vi "interp_3d.vi"(0 "prelookup_x":cluster{"frac":dbl, "num":u8}, 1 "prelookup_y":cluster{"frac":dbl, "num":u8}, 2 "z":dbl[][](array[numeric])) -> (7 "z":dbl)   [LabVIEW 2013]
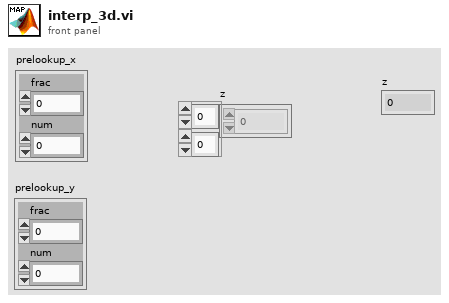
[diagram p1: front panel]
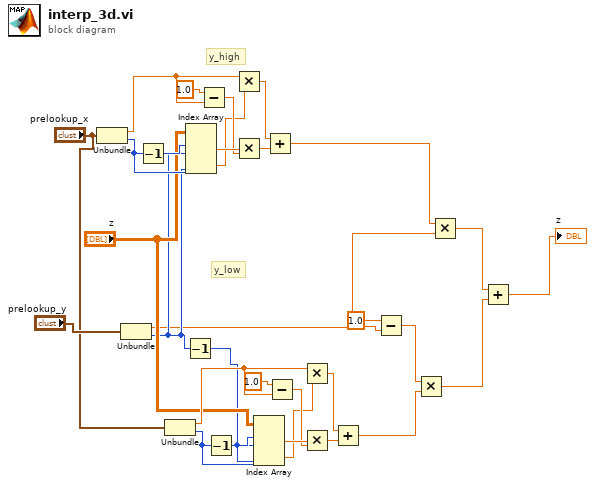
[diagram p0: block diagram]
diagram:
  # "y_low"
  # "y_high"
  n1 = Unbundle("prelookup_x") -> ("frac"=w30:dbl, "num"=w26:u8)
  n2 = Unbundle("prelookup_y") -> ("frac"=w2:dbl, "num"=w5:u8)
  n3 = Decrement(x=w26) -> (x-1=w27:u8)
  n4 = Unbundle("prelookup_x") -> ("frac"=w20:dbl, "num"=w16:u8)
  n5 = Decrement(x=w5) -> (x-1=w4:u8)
  n6 = Index Array(array="z", index (row) #1=w27, index (col) #1=w5, index (row) #2=w26, index (col) #2=w5) -> (element #1=w25:dbl, element #2=w23:dbl)
  n7 = Subtract(x=1.0, y=w30) -> (x-y=w24:dbl)
  n8 = Decrement(x=w16) -> (x-1=w17:u8)
  n9 = Multiply(x=w30, y=w23) -> (x*y=w29:dbl)
  n10 = Multiply(x=w25, y=w24) -> (x*y=w28:dbl)
  n11 = Index Array(array="z", index (row) #1=w17, index (col) #1=w4, index (row) #2=w16, index (col) #2=w4) -> (element #1=w15:dbl, element #2=w13:dbl)
  n12 = Add(x=w29, y=w28) -> (x+y=w9:dbl)
  n13 = Subtract(x=1.0, y=w20) -> (x-y=w14:dbl)
  n14 = Multiply(x=w20, y=w13) -> (x*y=w19:dbl)
  n15 = Multiply(x=w15, y=w14) -> (x*y=w18:dbl)
  n16 = Add(x=w19, y=w18) -> (x+y=w10:dbl)
  n17 = Subtract(x=1.0, y=w2) -> (x-y=w3:dbl)
  n18 = Multiply(x=w3, y=w10) -> (x*y=w7:dbl)
  n19 = Multiply(x=w9, y=w2) -> (x*y=w8:dbl)
  n20 = Add(x=w8, y=w7) -> (x+y=→"z":dbl)
